vi "Convert Volts to dBV array.vi"(4 "Volts":dbl[](array[numeric])) -> (1 "dBV":dbl[](array[numeric]))   [LabVIEW 2011]
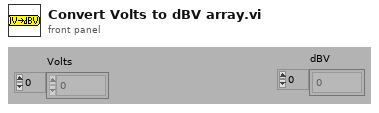
[diagram p1: front panel]
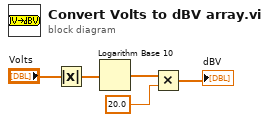
[diagram p0: block diagram]
diagram:
  n1 = Absolute Value(x="Volts") -> (abs(x)=w1:dbl[])
  n2 = Logarithm Base 10(1:w1) -> (0:w5:dbl[])
  n3 = Multiply(x=w5, y=20.0) -> (x*y=→"dBV":dbl[])
